vi "Find Class Method Reference.vi"(8 "error in":errorcluster, 9 "Method Name":string, 10 "Class Reference":refnum<vi>) -> (0 "error out":errorcluster, 1 "Method Reference":refnum<vi>)   [LabVIEW 2021, in "_Rename.lvlib"]
uses:
  _Rename.lvlib
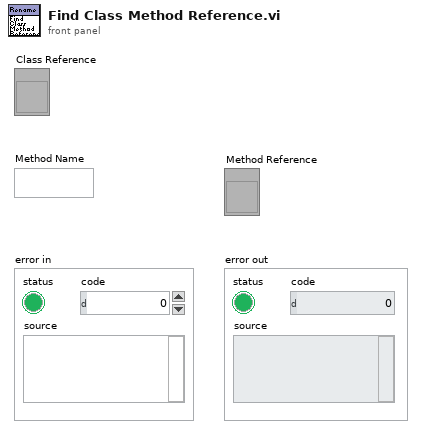
[diagram p1: front panel]
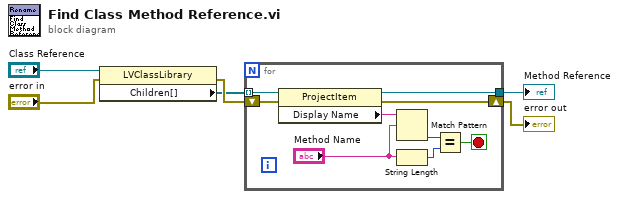
[diagram p0: block diagram]
diagram:
  n1 = property class="LVClassLibrary"(reference="Class Reference", error in="error in") -> (error out=w6:errorcluster, "Children[]"=w1:refnum<vi>[])  [unwired: 1 out]
  n2 = for {
    tunnel: w1 -> [w15] mode=indexing
    shift-right: [w13] -> w3
    shift-left: w6 -> [w14]
    tunnel: [w12] -> w2
    stop <- w10 stop-if-true
    n3 = property class="ProjectItem"(reference=w15, error in=w14) -> (reference out=w12:refnum<vi>, error out=w13:errorcluster, "Display Name"=w11:string)
    n4 = Match Pattern(string=w11, regular expression="Method Name") -> (offset past match=w9:i32)  [unwired: 1 in, 3 out]
    n5 = String Length(string="Method Name") -> (length=w8:i32)
    n6 = Equal?(x=w9, y=w8) -> (x = y?=w10:bool)
  }
  "Method Reference" <- w2
  "error out" <- w3
